vi "Update Tree.vi"(8 "error in (no error)":errorcluster, 11 "BuildServer in":refnum<class "BuildServer.lvclass">) -> (0 "error out":errorcluster, 3 "BuildServer out":refnum<class "BuildServer.lvclass">)   [LabVIEW 2017, in "BuildServer.lvlib" / "BuildServer.lvclass"]
uses:
  BuildServer.lvclass
  <vilib>/Ekim/LUT/LUT/LUT.lvclass
  BuildWorker/Classes/Task/Task.lvclass
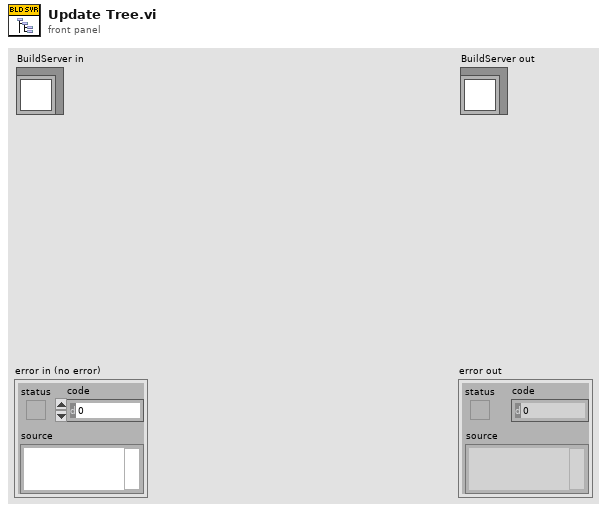
[diagram p1: front panel]
types:
  T1 = typedef "BuildServer.lvlib/BuildServer.lvclass/ProjectOrganization.ctl" = enum16{"Group by Project", "Group by Target", "Group by Type", "Group by Name"}
  T2 = cluster{cluster{"Properties:BuildSpec Name":string, i32}[]}[]
  T3 = cluster{cluster{"Properties:BuildSpec Name":string, i32}[]}
  T4 = cluster{"Properties:BuildSpec Name":string, i32}[]
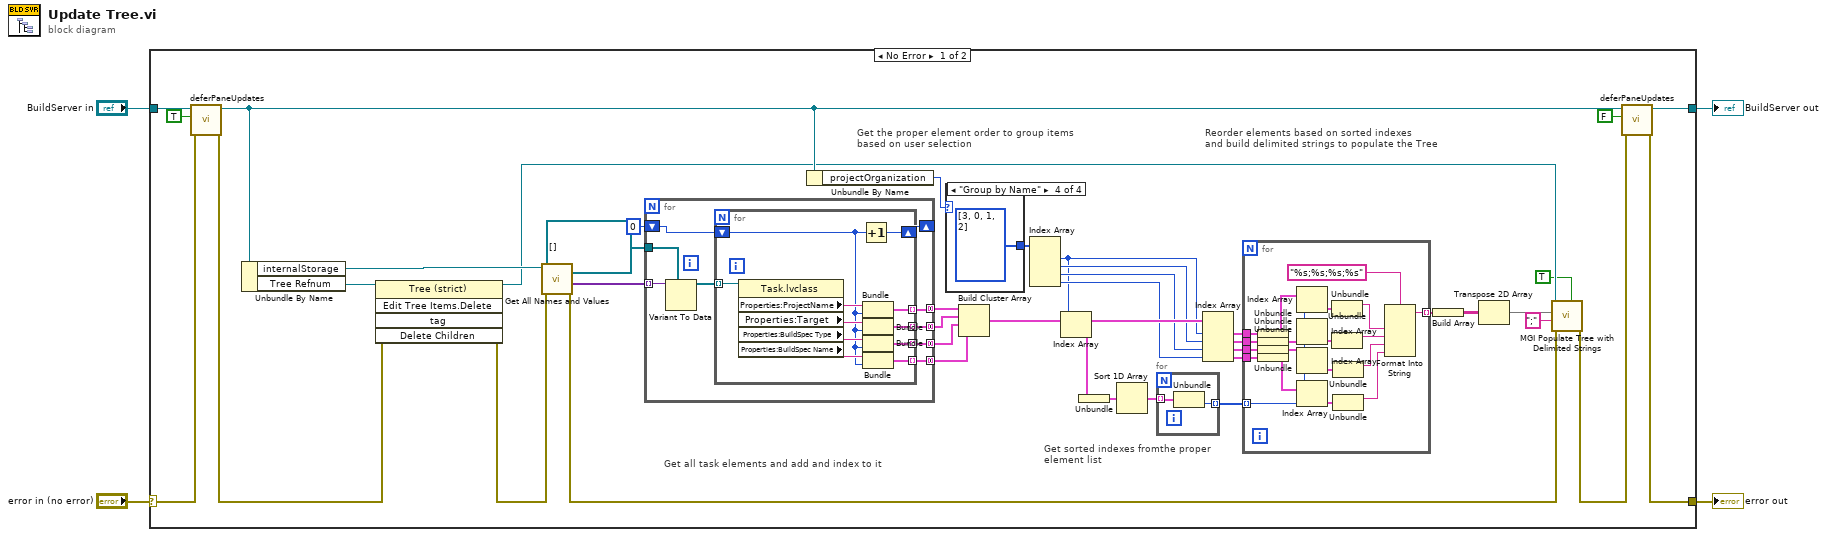
[diagram p0: block diagram]
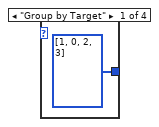
[diagram p2: hidden frame]
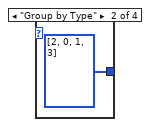
[diagram p3: hidden frame]
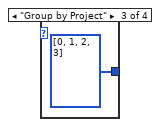
[diagram p4: hidden frame]
diagram:
  n1 = case shown="No Error" "error in (no error)" {
    selector: "error in (no error)" -> [w37 w92]
    tunnel: [w44 w92] -> w3
    tunnel: [w39 w91] -> w1
    tunnel: "BuildServer in" -> [w40 w91]
    frame No Error {
      # "Reorder elements based on sorted indexes\nand build delimited strings to populate the Tree"
      # "Get sorted indexes fromthe proper\nelement list"
      # "Get the proper element order to group items\nbased on user selection"
      # "Get all task elements and add and index to it"
      n2 = call "deferPaneUpdates.vi"("error in (no error)"=w37, "Defer Updates"=TRUE, "BuildServer in"=w40) -> ("error out"=w36:errorcluster, "BuildServer out"=w26:refnum<class "BuildServer.lvclass">)  [unwired: 7 in]
      n3 = Unbundle By Name(w26) -> ("internalStorage"=w43:refnum<class "LUT.lvclass">, "Tree Refnum"=w42:refnum<vi>)
      n4 = invoke class="Tree (strict)" method="Edit Tree Items.Delete"(reference=w42, error in=w36) -> (reference out=w23:refnum<vi>, error out=w41:errorcluster)  [unwired: 3 in, 3 out]
      n5 = call <vilib>:"Get All Names and Values.vi"("error in (no error)"=w41, "LUT in"=w43) -> ("error out"=w8:errorcluster, "Values"=w34:variant[])  [unwired: 6 in, 2 out]
      n6 = for {
        tunnel: w34 -> [w79] mode=indexing
        tunnel: refnum<class "Task.lvclass">[] [] -> [w78]
        tunnel: [w76] -> w27 mode=concatenating
        tunnel: [w75] -> w28 mode=concatenating
        tunnel: [w74] -> w29 mode=concatenating
        tunnel: [w73] -> w30 mode=concatenating
        shift-right: [w71] -> _
        shift-left: 0 -> [w72]
        n7 = Variant To Data(type=w78, Variant=w79) -> (data=w77:refnum<class "Task.lvclass">[])  [unwired: 1 in, 1 out]
        n8 = for {
          tunnel: w77 -> [w90] mode=indexing
          tunnel: [w85] -> w73 mode=indexing
          tunnel: [w84] -> w74 mode=indexing
          tunnel: [w83] -> w75 mode=indexing
          tunnel: [w82] -> w76 mode=indexing
          shift-right: [w80] -> w71
          shift-left: w72 -> [w81]
          n9 = property class="Task.lvclass"(reference=w90) -> ("Properties:ProjectName"=w86:string, "Properties:Target"=w87:string, "Properties:BuildSpec Type"=w88:string, "Properties:BuildSpec Name"=w89:string)  [unwired: 1 in, 2 out]
          n10 = Increment(x=w81) -> (x+1=w80:i32)
          n11 = Bundle("Properties:ProjectName"=w86, w81) -> (w85:cluster{"Properties:ProjectName":string, i32})  [unwired: 1 in]
          n12 = Bundle("Properties:Target"=w87, w81) -> (w84:cluster{"Properties:Target":string, i32})  [unwired: 1 in]
          n13 = Bundle("Properties:BuildSpec Type"=w88, w81) -> (w83:cluster{"Properties:BuildSpec Type":string, i32})  [unwired: 1 in]
          n14 = Bundle("Properties:BuildSpec Name"=w89, w81) -> (w82:cluster{"Properties:BuildSpec Name":string, i32})  [unwired: 1 in]
        }
      }
      n15 = Unbundle By Name(w26) -> ("projectOrganization"=w5:T1)
      n16 = case shown="\"Group by Name\"" w5 {
        tunnel: [i32[] [1, 0, 2, 3] ("index") i32[] [2, 0, 1, 3] ("index") i32[] [0, 1, 2, 3] ("index") i32[] [3, 0, 1, 2] ("index")] -> w19
        frame "Group by Target" {
        }
        frame "Group by Type" {
        }
        frame "Group by Project" {
        }
        frame "Group by Name" {
        }
      }
      n17 = Build Cluster Array(w30, w29, w28, w27) -> (w24:T2)
      n18 = Index Array(array=w19) -> (element #1=w6:i32, element #2=w18:i32, element #3=w17:i32, element #4=w16:i32)  [unwired: 4 in]
      n19 = Index Array(array=w24, index=w6) -> (element=w33:T3)
      n20 = Unbundle(w33) -> (w32:T4)
      n21 = Sort 1D Array(array=w32) -> (sorted array=w31:T4)
      n22 = for {
        tunnel: w31 -> [w70] mode=indexing
        tunnel: [w69] -> w25 mode=indexing
        n23 = Unbundle(w70) -> (w69:i32)  [unwired: 1 out]
      }
      n24 = Index Array(array=w24, index #1=w6, index #2=w18, index #3=w17, index #4=w16) -> (element #1=w20:T3, element #2=w15:T3, element #3=w14:T3, element #4=w13:T3)
      n25 = for {
        tunnel: w25 -> [w57] mode=indexing
        tunnel: w20 -> [w64]
        tunnel: w15 -> [w60]
        tunnel: w14 -> [w59]
        tunnel: w13 -> [w58]
        tunnel: [w46] -> w12 mode=indexing
        n26 = Unbundle(w64) -> (w63:T4)
        n27 = Unbundle(w60) -> (w61:T4)
        n28 = Unbundle(w59) -> (w56:T4)
        n29 = Unbundle(w58) -> (w55:T4)
        n30 = Index Array(array=w63, index=w57) -> (element=w62:cluster{"Properties:BuildSpec Name":string, i32})
        n31 = Index Array(array=w61, index=w57) -> (element=w52:cluster{"Properties:BuildSpec Name":string, i32})
        n32 = Index Array(array=w56, index=w57) -> (element=w53:cluster{"Properties:BuildSpec Name":string, i32})
        n33 = Index Array(array=w55, index=w57) -> (element=w54:cluster{"Properties:BuildSpec Name":string, i32})
        n34 = Unbundle(w62) -> ("Properties:BuildSpec Name"=w51:string)  [unwired: 1 out]
        n35 = Unbundle(w52) -> ("Properties:BuildSpec Name"=w50:string)  [unwired: 1 out]
        n36 = Unbundle(w53) -> ("Properties:BuildSpec Name"=w49:string)  [unwired: 1 out]
        n37 = Unbundle(w54) -> ("Properties:BuildSpec Name"=w48:string)  [unwired: 1 out]
        n38 = Format Into String(format string="%s;%s;%s;%s", w51, w50, w49, w48) -> (resulting string=w46:string)  [unwired: 2 in, 1 out]
      }
      n39 = Build Array(w12) -> (w11:string[][])
      n40 = Transpose 2D Array(2D array=w11) -> (transposed array=w10:string[][])
      n41 = call <userlib>:"MGI Populate Tree with Delimited Strings.vi"("Use Child Only?"=TRUE, "error in (no error)"=w8, "Delimiter"=";", "Items (Delimited)"=w10, "Tree Control"=w23) -> ("error out"=w7:errorcluster)  [unwired: 4 in, 2 out]
      n42 = call "deferPaneUpdates.vi"("error in (no error)"=w7, "Defer Updates"=FALSE, "BuildServer in"=w26) -> ("error out"=w44:errorcluster, "BuildServer out"=w39:refnum<class "BuildServer.lvclass">)  [unwired: 7 in]
    }
    frame Error {
    }
  }
  "error out" <- w3
  "BuildServer out" <- w1
